vi "ABFImport_ReadChannel.vi"(8 "error in (no error)":errorcluster, 10 "channel number":i32, 11 "reference number":i32) -> (0 "error out":errorcluster, 2 "signal":sgl[](array[numeric]), 3 "reference out":i32)   [LabVIEW 2017]
uses:
  LV_ABFIO.dll
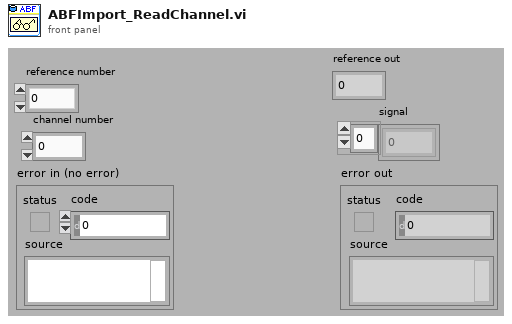
[diagram p1: front panel]
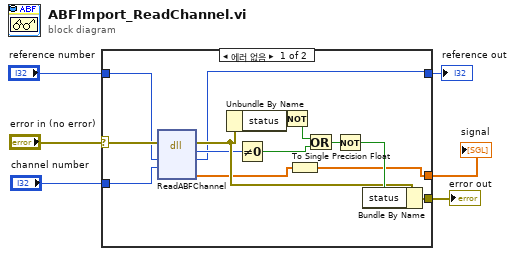
[diagram p0: block diagram]
diagram:
  n1 = case shown="에러 없음" "error in (no error)" {
    selector: "error in (no error)" -> [w14 w22]
    tunnel: [w15 w22] -> w5
    tunnel: "reference number" -> [w11 w21]
    tunnel: [w10 w21] -> w3
    tunnel: "channel number" -> [w9 _]
    tunnel: [w7 _] -> w1
    frame No Error {
      n2 = dll-call lib="C:/Users/KimYG/Application/Solution Package/APIs/LV_ABFIO.dll" fn="ReadABFChannel"(error in=w14, "arg3"=w11, "arg2"=w9) -> (error out=w13:errorcluster, "return type"=w12:i32, "arg3"=w10:i32, "arg4"=w8:dbl[])  [unwired: 4 in, 1 out]
      n3 = Unbundle By Name(w13) -> ("status"=w20:bool)
      n4 = Not Equal To 0?(x=w12) -> (x != 0?=w18:bool)
      n5 = Not(x=w20) -> (.not. x?=w19:bool)
      n6 = To Single Precision Float(number=w8) -> (single precision float=w7:sgl[])
      n7 = Or(x=w19, y=w18) -> (x .or. y?=w17:bool)
      n8 = Not(x=w17) -> (.not. x?=w16:bool)
      n9 = Bundle By Name(cluster=w13, "status"=w16) -> (w15:errorcluster)
    }
    frame Error {
    }
  }
  "error out" <- w5
  "reference out" <- w3
  "signal" <- w1
